vi "Calculate_ON_OFF_samples.vi"(10 "Duty cycle":dbl, 11 "Step samples":dbl) -> (2 "OFF samples":dbl, 3 "ON samples":dbl)   [LabVIEW 2016]
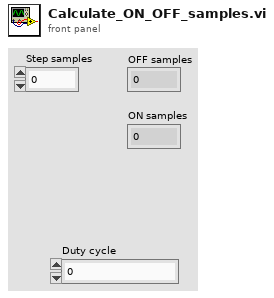
[diagram p1: front panel]
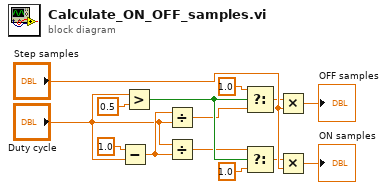
[diagram p0: block diagram]
diagram:
  n1 = Subtract(x=1.0, y="Duty cycle") -> (x-y=w4:dbl)
  n2 = Greater?(x="Duty cycle", y=0.5) -> (0:w14:bool)
  n3 = Divide(x=w4, y="Duty cycle") -> (x/y=w8:dbl)
  n4 = Divide(x="Duty cycle", y=w4) -> (x/y=w5:dbl)
  n5 = Select(t=1.0, s=w14, f=w8) -> (s? t:f=w10:dbl)
  n6 = Select(t=w5, s=w14, f=1.0) -> (s? t:f=w9:dbl)
  n7 = Multiply(x=w10, y="Step samples") -> (x*y=→"OFF samples":dbl)
  n8 = Multiply(x=w9, y="Step samples") -> (x*y=→"ON samples":dbl)
